vi "Poly_fit.vi"(1 "Input":dbl, 2 "Parameters":dbl[](array[numeric])) -> (0 "Output":dbl)   [LabVIEW 2016]
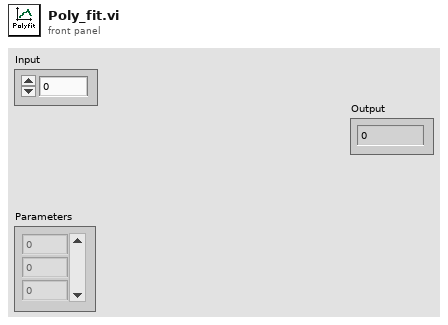
[diagram p1: front panel]
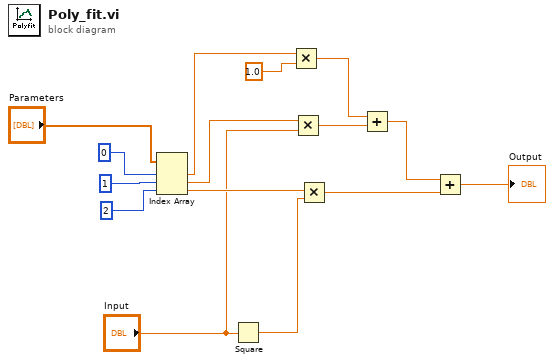
[diagram p0: block diagram]
diagram:
  n1 = Index Array(array="Parameters", index #1=0 ("index"), index #2=1 ("index"), index #3=2 ("index")) -> (element #1=w12:dbl, element #2=w10:dbl, element #3=w9:dbl)
  n2 = Square(x="Input") -> (x^2=w7:dbl)
  n3 = Multiply(x=w12, y=1.0) -> (x*y=w6:dbl)
  n4 = Multiply(x=w10, y="Input") -> (x*y=w5:dbl)
  n5 = Multiply(x=w9, y=w7) -> (x*y=w4:dbl)
  n6 = Add(x=w6, y=w5) -> (x+y=w3:dbl)
  n7 = Add(x=w3, y=w4) -> (x+y=→"Output":dbl)
